vi "Agilent SNA Initialize.vi"(8 "error in (no error)":errorcluster, 10 "Query Instrument? (T)":bool=TRUE, 11 "Configuration":T3={"BusType"=enum."GPIB", "GPIB Bus"=0, "GPIB Address"=16, "Pass Through Address"=19, "IP"=0, "SCIL Address"=16, "COM"=1, "Baud Rate"=enum."9600", "USB Device"=0, "Instrument S\\N"=""} {"USB Device" max=31 step=1}) -> (0 "error out":errorcluster {"code" format="%.0x"}, 1 "*IDN? String":string, 3 "VISA Resource Name":T2, 5 "Agilent SNA & SWP":T1)   [LabVIEW 2011]
uses:
  SNA Configuration.ctl
  TypeDefs/Agilent SNA VISA.ctl
  TypeDefs/Agilent SNA Instrument Info.ctl
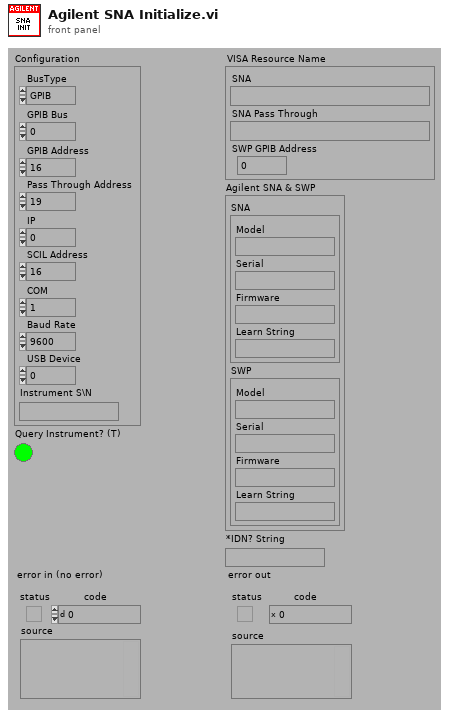
[diagram p1: front panel]
types:
  T1 = typedef "Agilent SNA Instrument Info.ctl" = cluster{"SNA":cluster{"Model":string, "Serial":string, "Firmware":string, "Learn String":string}, "SWP":cluster{"Model":string, "Serial":string, "Firmware":string, "Learn String":string}}
  T2 = typedef "Agilent SNA VISA.ctl" = cluster{"SNA":refnum<visa-resource-name>, "SNA Pass Through":refnum<visa-resource-name>, "SWP GPIB Address":i32}
  T3 = typedef "SNA Configuration.ctl" = cluster{"BusType":enum32{"GPIB", "LAN/IP", "Serial", "USB"}, "GPIB Bus":i32, "GPIB Address":i32, "Pass Through Address":i32, "IP":u32, "SCIL Address":i32, "COM":i32, "Baud Rate":enum32{"300", "600", "1200", "2400", "4800", "9600"}, "USB Device":i32, "Instrument S\\N":string}
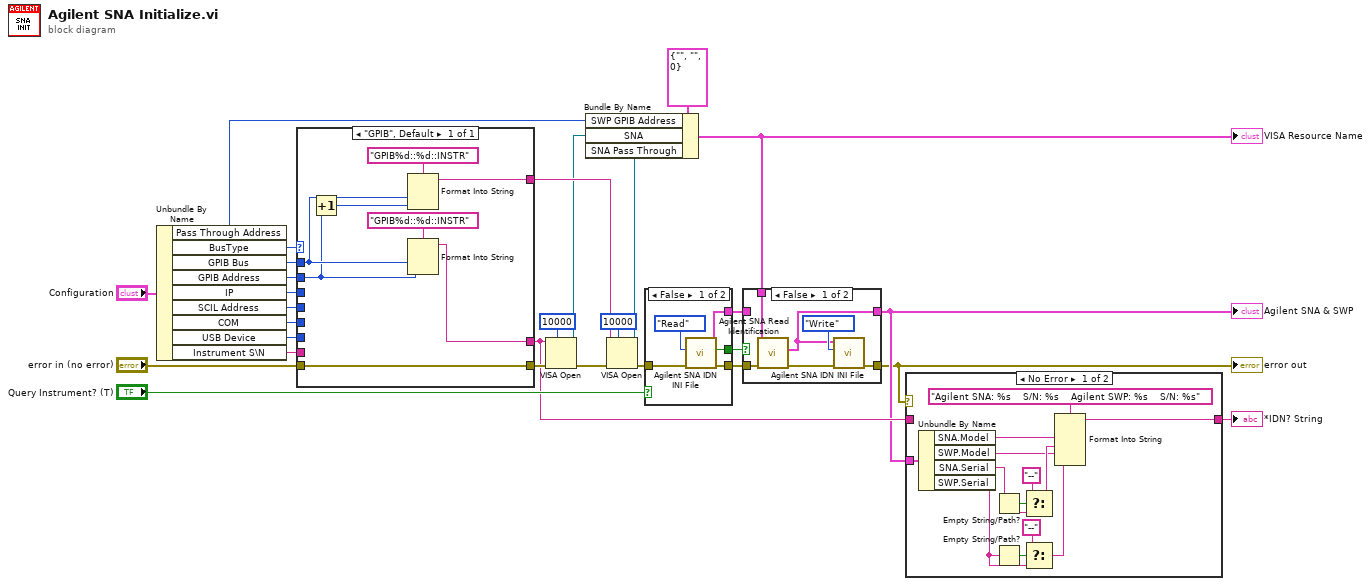
[diagram p0: block diagram]
diagram:
  n1 = Unbundle By Name("Configuration") -> ("Pass Through Address"=w10:i32, "BusType"=w27:enum32{"GPIB", "LAN/IP", "Serial", "USB"}, "GPIB Bus"=w26:i32, "GPIB Address"=w25:i32, "IP"=w23:u32, "SCIL Address"=w18:i32, "COM"=w24:i32, "USB Device"=w22:i32, "Instrument S\\N"=w19:string)
  n2 = case shown="\"GPIB\", Default" w27 {
    tunnel: "error in (no error)" -> [w36]
    tunnel: w26 -> [w33]
    tunnel: w25 -> [w31]
    tunnel: [w35] -> w8
    tunnel: [w36] -> w20
    tunnel: w24 -> [_]
    tunnel: w23 -> [_]
    tunnel: w22 -> [_]
    tunnel: w19 -> [_]
    tunnel: w18 -> [_]
    tunnel: [w30] -> w14
    frame "GPIB", Default {
      n3 = Increment(x=w31) -> (x+1=w32:i32)
      n4 = Format Into String(format string="GPIB%d::%d::INSTR", w33, w32) -> (resulting string=w30:string)  [unwired: 2 in, 1 out]
      n5 = Format Into String(format string="GPIB%d::%d::INSTR", w33, w31) -> (resulting string=w35:string)  [unwired: 2 in, 1 out]
    }
  }
  n6 = VISA Open(timeout (0)=u32 10000 ("VISA Open timeout (0)"), error in (no error)=w20, VISA resource name=w8) -> (VISA resource name=w12:refnum<visa-resource-name>, error out=w16:errorcluster)  [unwired: 2 out]
  n7 = VISA Open(timeout (0)=u32 10000 ("VISA Open timeout (0)"), error in (no error)=w16, VISA resource name=w14) -> (VISA resource name=w11:refnum<visa-resource-name>, error out=w15:errorcluster)  [unwired: 2 out]
  n8 = Bundle By Name(cluster=T2 {"SNA"="", "SNA Pass Through"="", "SWP GPIB Address"=0} ("VISA Resource Names"), "SWP GPIB Address"=w10, "SNA"=w12, "SNA Pass Through"=w11) -> (w1:T2)
  "VISA Resource Name" <- w1
  n9 = case shown="False" "Query Instrument? (T)" {
    tunnel: w15 -> [w42 w43]
    tunnel: [w41 w43] -> w6
    tunnel: [w39 _] -> w5
    tunnel: [w38 _] -> w3
    frame False {
      n10 = call "Agilent SNA IDN INI File.vi"("error in (no error)"=w42, "Operation"=enum16{"Read", "Write", "Clear"}."Read") -> ("error out"=w41:errorcluster, "Found?"=w38:bool, "Instrument Info"=w39:T1)  [unwired: 1 in, 6 out]
    }
    frame True {
    }
  }
  n11 = case shown="False" w3 {
    tunnel: w1 -> [w49 _]
    tunnel: w6 -> [w48 w50]
    tunnel: [w45 w50] -> w2
    tunnel: w5 -> [_ w51]
    tunnel: [w44 w51] -> w4
    frame False {
      n12 = call "Agilent SNA Read Identification.vi"("error in (no error)"=w48, "VISA Resource Names"=w49) -> ("error out"=w46:errorcluster, "Instrument Info"=w44:T1)  [unwired: 8 out]
      n13 = call "Agilent SNA IDN INI File.vi"("error in (no error)"=w46, "Operation"=enum16{"Read", "Write", "Clear"}."Write", "Instrument Info"=w44) -> ("error out"=w45:errorcluster)  [unwired: 8 out]
    }
    frame True {
    }
  }
  "error out" <- w2
  "Agilent SNA & SWP" <- w4
  n14 = case shown="No Error" w2 {
    tunnel: [w64 w65] -> w7
    tunnel: w8 -> [_ w65]
    tunnel: w4 -> [w56 _]
    frame No Error {
      n15 = Unbundle By Name(w56) -> ("SNA.Model"=w55:string, "SWP.Model"=w54:string, "SNA.Serial"=w53:string, "SWP.Serial"=w52:string)
      n16 = Empty String/Path?(string/path=w53) -> (empty?=w63:bool)
      n17 = Empty String/Path?(string/path=w52) -> (empty?=w58:bool)
      n18 = Select(t="--", s=w63, f=w53) -> (s? t:f=w61:string)
      n19 = Select(t="--", s=w58, f=w52) -> (s? t:f=w57:string)
      n20 = Format Into String(format string="Agilent SNA: %s    S/N: %s    Agilent SWP: %s    S/N: %s" ("Return Model and Serial #"), w55, w61, w54, w57) -> (resulting string=w64:string)  [unwired: 2 in, 1 out]
    }
    frame Error {
    }
  }
  "*IDN? String" <- w7
